vi "test15.1-MappingRelationshipByLocalRegistration_WIthSubscriberName_State.vi"(8 "error in (no error)":errorcluster, 11 "TestCase in":refnum<class "testcase-CSMBroadcast.lvclass">) -> (0 "error out":errorcluster, 3 "TestCase out":refnum<class "testcase-CSMBroadcast.lvclass">)   [LabVIEW 2017, in "testcase-CSMBroadcast.lvclass"]
uses:
  testcase-CSMBroadcast.lvclass
  caa41fc0-4920-4570-a7eb-0567c3b7bd6c.vi
  <vilib>/addons/_JKI Toolkits/VI Tester/TestCase.llb/TestCase.lvclass
  src/user.lib/_NEVSTOP/Communicable State Machine(CSM)/Communicable State Machine.lvlib
  CSM/CSM-Testcase.lvlib
  C:/Program Files (x86)/National Instruments/LabVIEW 2017/vi.lib/addons/_JKI Toolkits/VI Tester/TestCase.llb/TestCase.lvclass
panel:
  out "Loop Count":i32
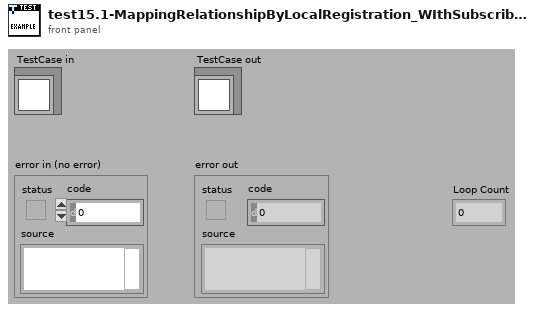
[diagram p1: front panel]
types:
  T1 = cluster{"Status":string, "Source CSM":string, "Target CSM":string, "Target API":string}[]
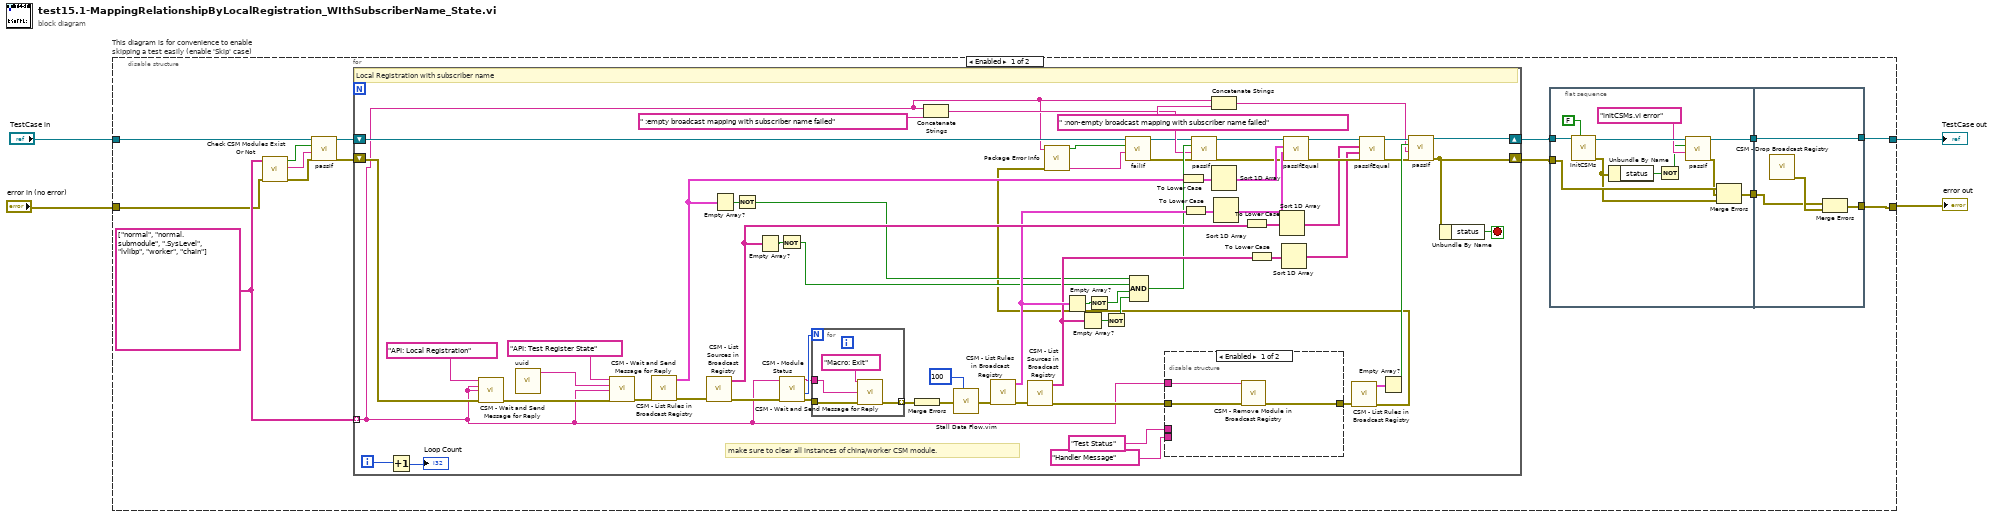
[diagram p0: block diagram]
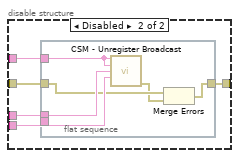
[diagram p2: hidden frame]
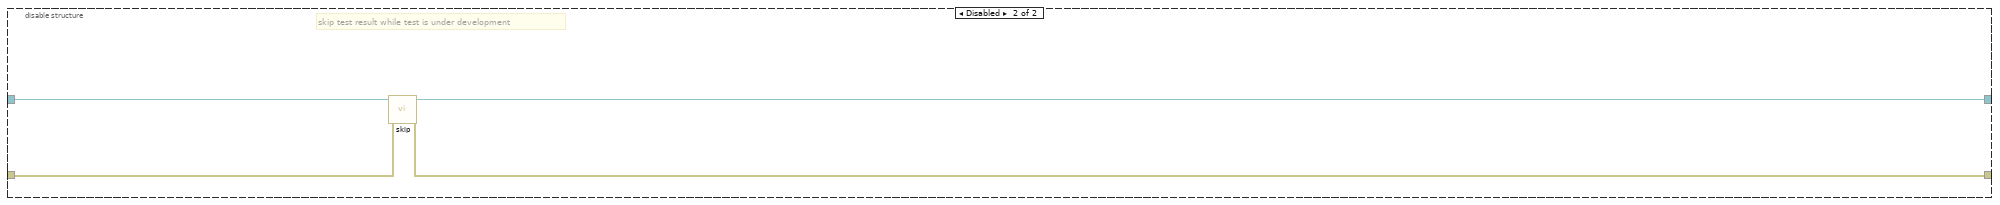
[diagram p3: hidden frame]
diagram:
  n1 = disable-structure "This diagram is for convenience to enable skipping a test easily (enable 'Skip' case)" shown="Enabled" {
    disable-tunnel: "TestCase in" -> [w14 w120]
    disable-tunnel: [w6 w118] -> w1
    disable-tunnel: [w5 w119] -> w3
    disable-tunnel: "error in (no error)" -> [w12 w117]
    frame Enabled {
      w15 = string[] ["normal", "normal.submodule", ".SysLevel", "lvlibp", "worker", "chain"]
      n2 = call "Check CSM Modules Exist Or Not.vi"("error in"=w12, "CSM names in"=w15) -> ("error out"=w16:errorcluster, "Debug string"=w17:string, "All Modules Exist?"=w18:bool)  [unwired: 7 in]
      n3 = call-dynamic "passIf.vi"("error in (no error)"=w16, "message (\"\")"=w17, "pass"=w18, "TestCase in"=w14) -> ("error out"=w11:errorcluster, "TestCase out"=w13:refnum<class "testcase-CSMBroadcast.lvclass">)  [unwired: 6 in]
      n4 = for {
        tunnel: w15 -> [w36] mode=indexing
        shift-right: [w58] -> w8
        shift-left: w13 -> [w39]
        shift-right: [w59] -> w7
        shift-left: w11 -> [w49]
        i -> [w79]
        stop <- w92 stop-if-true
        # "make sure to clear all instances of china/worker CSM module."
        # "Local Registration with subscriber name"
        n5 = Increment(x=w79) -> (x+1=→"Loop Count":i32)
        n6 = call "CSM - Wait and Send Message for Reply.vi"("State"="API: Local Registration", "Arguments (\"\")"=w36, "Target Module"=w36, "Error In (No Error)"=w49) -> ("error out"=w97:errorcluster)  [unwired: 8 in, 3 out]
        n7 = call "uuid.vi"() -> ("UUID"=w95:string)  [unwired: 11 in]
        n8 = call "CSM - Wait and Send Message for Reply.vi"("State"="API: Test Register State", "Arguments (\"\")"=w95, "Target Module"=w36, "Error In (No Error)"=w97) -> ("error out"=w94:errorcluster)  [unwired: 8 in, 3 out]
        n9 = call "CSM - List Rules in Broadcast Registry.vi"("error in (no error)"=w94) -> ("error out"=w91:errorcluster, "Rule Entries"=w77:T1)  [unwired: 8 in, 1 out]
        n10 = call "CSM - List Sources in Broadcast Registry.vi"("error in (no error)"=w91) -> ("error out"=w54:errorcluster, "Broadcast Names"=w74:string[])  [unwired: 9 in]
        n11 = Empty Array?(array=w77) -> (empty?=w76:bool)
        n12 = Not(x=w76) -> (.not. x?=w69:bool)
        n13 = Empty Array?(array=w74) -> (empty?=w75:bool)
        n14 = Not(x=w75) -> (.not. x?=w68:bool)
        n15 = call "CSM - Module Status.vi"("Error In"=w54, "CSM Name"=w36) -> ("error out"=w55:errorcluster, "#Nodes"=w57:i32, "CSM Name (Dup)"=w56:string)  [unwired: 5 in, 2 out]
        n16 = for {
          N: w57 -> [_]
          tunnel: w56 -> [w100]
          tunnel: w55 -> [w99]
          tunnel: [w101] -> w93 mode=indexing
          n17 = call "CSM - Wait and Send Message for Reply.vi"("State"="Macro: Exit", "Target Module"=w100, "Error In (No Error)"=w99) -> ("error out"=w101:errorcluster)  [unwired: 9 in, 3 out]
        }
        n18 = Merge Errors(w93) -> (w43:errorcluster)
        n19 = Concatenate Strings(w36, " :empty broadcast mapping with subscriber name failed" ("string")) -> (w45:string)
        n20 = call "Stall Data Flow.vim"("value in"=w43, "milliseconds to wait"=u32 100) -> ("value out"=w42:errorcluster)  [unwired: 1 out]
        n21 = call "CSM - List Rules in Broadcast Registry.vi"("error in (no error)"=w42) -> ("error out"=w90:errorcluster, "Rule Entries"=w72:T1)  [unwired: 8 in, 1 out]
        n22 = call "CSM - List Sources in Broadcast Registry.vi"("error in (no error)"=w90) -> ("error out"=w65:errorcluster, "Broadcast Names"=w70:string[])  [unwired: 9 in]
        n23 = Empty Array?(array=w72) -> (empty?=w73:bool)
        n24 = Empty Array?(array=w70) -> (empty?=w71:bool)
        n25 = Not(x=w73) -> (.not. x?=w67:bool)
        n26 = Not(x=w71) -> (.not. x?=w66:bool)
        n27 = Compound Arithmetic op=AND(w69, w68, w67, w66) -> (w48:bool)
        n28 = disable-structure shown="Enabled" {
          disable-tunnel: w65 -> [w105 w107]
          disable-tunnel: [w104 w106] -> w62
          disable-tunnel: w36 -> [w103 w108]
          disable-tunnel: "Test Status" ("Status") -> [_ w110]
          disable-tunnel: "Handler Message" ("Response Message (If \"\", Same as Source Message)") -> [_ w109]
          frame Enabled {
            n29 = call "CSM - Remove Module in Broadcast Registry.vi"("CSM Name"=w103, "Error In"=w105) -> ("error out"=w104:errorcluster)  [unwired: 12 in, 1 out]
          }
          frame Disabled {
            n30 = flat-sequence {
              tunnel: w110 -> [w116]
              tunnel: w109 -> [w115]
              tunnel: w108 -> [w114]
              tunnel: w107 -> [w113]
              tunnel: [w111] -> w106
              frame #0 {
                n31 = call "CSM - Unregister Broadcast.vi"("CSM Name(Empty for Broadcast Event)"=w114, "Source CSM Name (* as Default)"=w114, "Trigger"=w116, "API (\"*\" as Default)"=w115) -> ("error out"=w112:errorcluster)  [unwired: 10 in, 1 out]
                n32 = Merge Errors(w113, w112) -> (w111:errorcluster)
              }
            }
          }
        }
        n33 = To Lower Case(string=w77) -> (all lower case string=w89:T1)
        n34 = To Lower Case(string=w72) -> (all lower case string=w88:T1)
        n35 = Concatenate Strings(w36, " :non-empty broadcast mapping with subscriber name failed" ("string")) -> (w44:string)
        n36 = Sort 1D Array(array=w89) -> (sorted array=w87:T1)
        n37 = Sort 1D Array(array=w88) -> (sorted array=w86:T1)
        n38 = To Lower Case(string=w74) -> (all lower case string=w83:string[])
        n39 = To Lower Case(string=w70) -> (all lower case string=w82:string[])
        n40 = Sort 1D Array(array=w83) -> (sorted array=w81:string[])
        n41 = Sort 1D Array(array=w82) -> (sorted array=w80:string[])
        n42 = call "CSM - List Rules in Broadcast Registry.vi"("error in (no error)"=w62) -> ("error out"=w37:errorcluster, "Rule Entries"=w61:T1)  [unwired: 8 in, 1 out]
        n43 = call "Package Error Info.vi"("error in"=w37, "String in"=w36) -> ("packed error info out"=w34:string, "error status"=w35:bool)  [unwired: 8 in]
        n44 = call-dynamic "failIf.vi"("message (\"\")"=w34, "fail"=w35, "TestCase in"=w39) -> ("error out"=w38:errorcluster, "TestCase out"=w40:refnum<class "testcase-CSMBroadcast.lvclass">)  [unwired: 7 in]
        n45 = call-dynamic "passIf.vi"("error in (no error)"=w38, "message (\"\")"=w45, "pass"=w48, "TestCase in"=w40) -> ("error out"=w50:errorcluster, "TestCase out"=w51:refnum<class "testcase-CSMBroadcast.lvclass">)  [unwired: 6 in]
        n46 = call-dynamic "passIfEqual.vi"("error in (no error)"=w50, "y"=w86, "x"=w87, "TestCase in"=w51) -> ("error out"=w84:errorcluster, "TestCase out"=w85:refnum<class "testcase-CSMBroadcast.lvclass">)  [unwired: 6 in]
        n47 = call-dynamic "passIfEqual.vi"("error in (no error)"=w84, "y"=w80, "x"=w81, "TestCase in"=w85) -> ("error out"=w52:errorcluster, "TestCase out"=w53:refnum<class "testcase-CSMBroadcast.lvclass">)  [unwired: 6 in]
        n48 = Empty Array?(array=w61) -> (empty?=w60:bool)
        n49 = call-dynamic "passIf.vi"("error in (no error)"=w52, "message (\"\")"=w44, "pass"=w60, "TestCase in"=w53) -> ("error out"=w59:errorcluster, "TestCase out"=w58:refnum<class "testcase-CSMBroadcast.lvclass">)  [unwired: 6 in]
        n50 = Unbundle By Name(w59) -> ("status"=w92:bool)
      }
      n51 = flat-sequence {
        tunnel: w8 -> [w29]
        tunnel: [w26] -> w10
        tunnel: w7 -> [w23]
        tunnel: [w20] -> w9
        tunnel: w10 -> [w32]
        tunnel: [w32] -> w6
        tunnel: [w31] -> w5
        tunnel: w9 -> [w30]
        frame #0 {
          n52 = call "InitCSMs.vi"("Enable building lvlibp?"=FALSE, "testcase-CSMStatus in"=w29) -> ("error out"=w21:errorcluster, "testcase-CSMStatus out"=w27:refnum<class "testcase-CSMBroadcast.lvclass">)  [unwired: 8 in]
          n53 = Unbundle By Name(w21) -> ("status"=w25:bool)
          n54 = Not(x=w25) -> (.not. x?=w19:bool)
          n55 = call-dynamic "passIf.vi"("message (\"\")"="initCSMs.vi error" ("message (\"\")"), "pass"=w19, "TestCase in"=w27) -> ("error out"=w22:errorcluster, "TestCase out"=w26:refnum<class "testcase-CSMBroadcast.lvclass">)  [unwired: 7 in]
          n56 = Merge Errors(w23, w22, w21) -> (w20:errorcluster)
        }
        frame #1 {
          n57 = call "CSM - Drop Broadcast Registry.vi"() -> ("error out"=w33:errorcluster)  [unwired: 15 in]
          n58 = Merge Errors(w30, w33) -> (w31:errorcluster)
        }
      }
    }
    frame Disabled {
      # "skip test result while test is under development"
      n59 = call <vilib>:"skip.vi"("error in (no error)"=w117, "TestCase in"=w120) -> ("error out"=w119:errorcluster, "TestCase out"=w118:refnum<class "testcase-CSMBroadcast.lvclass">)  [unwired: 8 in]
    }
  }
  "error out" <- w3
  "TestCase out" <- w1
